vi "Lookup Forwards.vi"(8 "error in (no error)":errorcluster, 11 "Data Processor Module in":refnum<class "Data Processor Module.lvclass">) -> (0 "error out":errorcluster, 3 "Data Processor Module out":refnum<class "Data Processor Module.lvclass">)   [LabVIEW 2020, in "VolatusData.lvlib" / "Data Processor Module.lvclass"]
uses:
  Data Processor Module.lvclass
  Data Processor Module.lvclass/Data Processor Module.ctl
  Volatus/Module/Module.lvclass
  Volatus/VolatusAPI/VolatusAPI.lvclass
  Volatus/Module Identity/Module Identity.lvclass
  C:/dev/lv20CE/relink/lv-volatus/Volatus/Module/Module.lvclass
  C:/dev/lv20CE/relink/lv-volatus/VolatusData/Data Processor Module/Data Processor Module.lvclass
  C:/dev/lv20CE/relink/lv-volatus/Volatus/Module Identity/Module Identity.lvclass
  C:/dev/lv20CE/relink/lv-volatus/Volatus/Identity/Identity.lvclass
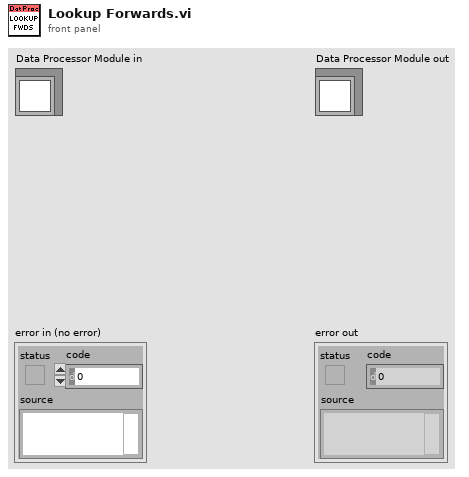
[diagram p1: front panel]
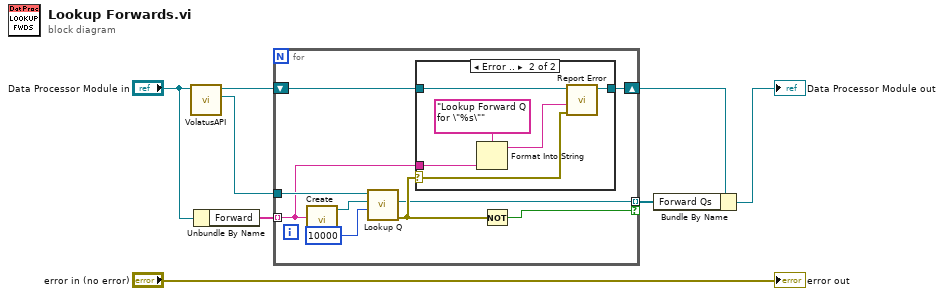
[diagram p0: block diagram]
diagram:
  n1 = call "VolatusAPI.vi"("Module in"="Data Processor Module in") -> ("VolatusAPI"=w7:refnum<class "VolatusAPI.lvclass">, "Module out"=w4:refnum<class "Data Processor Module.lvclass">)  [unwired: 9 in]
  n2 = Unbundle By Name("Data Processor Module in") -> ("Forward"=w5:string[])
  n3 = for {
    tunnel: w7 -> [w16]
    tunnel: w5 -> [w9] mode=indexing
    shift-right: [w12] -> w3
    shift-left: w4 -> [w13]
    tunnel: [w11] -> w2 mode=indexing if=w10
    n4 = call "Create.vi"("ID"=w9) -> ("Module Identity out"=w15:refnum<class "Module Identity.lvclass">)  [unwired: 10 in]
    n5 = call "Lookup Q.vi"("Timeout ms (0)"=10000, "Identity"=w15, "VolatusAPI in"=w16) -> ("error out"=w17:errorcluster, "MessageQ"=w11:refnum<class "MessageQ.lvclass">)  [unwired: 6 in, 1 out]
    n6 = case shown="Error .." w17 {
      selector: w17 -> [_ w22]
      tunnel: w13 -> [w18 w24]
      tunnel: [w18 w23] -> w12
      tunnel: w9 -> [_ w19]
      frame No Error {
      }
      frame Error {
        n7 = Format Into String(format string="Lookup Forward Q for \"%s\"", w19) -> (resulting string=w20:string)  [unwired: 2 in, 1 out]
        n8 = call "Report Error.vi"("error in (no error)"=w22, "Message (None)"=w20, "Module in"=w24) -> ("Module out"=w23:refnum<class "Data Processor Module.lvclass">)  [unwired: 7 in, 1 out]
      }
    }
    n9 = Not(x=w17) -> (.not. x?=w10:bool)
  }
  n10 = Bundle By Name(cluster=w3, "Forward Qs"=w2) -> (→"Data Processor Module out":refnum<class "Data Processor Module.lvclass">)
  "error out" <- "error in (no error)"
